vi "Field Centric Teleop Emulator.vi"(10 "Current Heading":dbl, 11 "device ID":refnum<k1>) -> (3 "Robot Velocities":T1)   [LabVIEW 2020]
uses:
  <vilib>/Analysis/NI_AALPro.lvlib
  <vilib>/Analysis/coordinate.llb/2D Cartesian Coordinate Rotation (Scalar).vi
  Drive/Implementation/Robot Velocities.ctl
panel:
  in  "Max Velocities":cluster{"vx":dbl, "vy":dbl, "w":dbl}={"vx"=10.0, "vy"=10.0, "w"=180.0}
  in  "Deadband":dbl=0.1
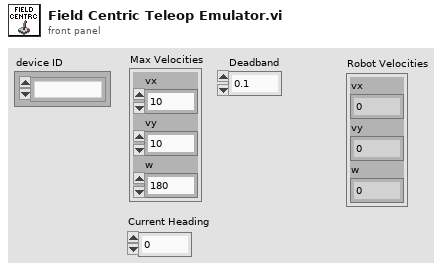
[diagram p1: front panel]
types:
  T1 = typedef "Robot Velocities.ctl" = cluster{"vx":dbl, "vy":dbl, "w":dbl}
  T2 = cluster{"X axis":i32, "Y axis":i32, "Z axis":i32, "X axis rotation":i32, "Y axis rotation":i32, "Z axis rotation":i32, "U axis":i32, "V axis":i32}
  T3 = cluster{"X axis":dbl, "Y axis":dbl, "Z axis":dbl, "X axis rotation":dbl, "Y axis rotation":dbl, "Z axis rotation":dbl, "U axis":dbl, "V axis":dbl}
  T4 = cluster{"X axis":dbl, dbl, "X axis rotation":dbl}
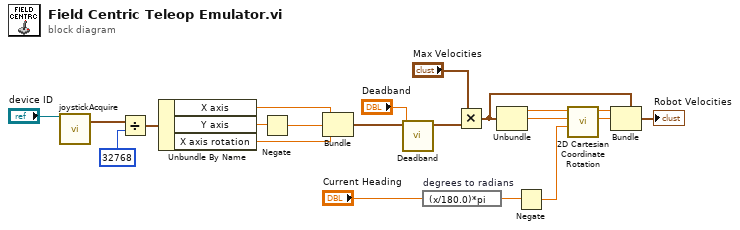
[diagram p0: block diagram]
diagram:
  n1 = call <vilib>:"joystickAcquire.vi"("device ID"="device ID") -> ("axis info"=w17:T2)  [unwired: 14 in, 4 out]
  n2 = Divide(x=w17, y=32768 ("X axis")) -> (x/y=w15:T3)
  n3 = Unbundle By Name(w15) -> ("X axis"=w13:dbl, "Y axis"=w11:dbl, "X axis rotation"=w12:dbl)
  n4 = Negate(x=w11) -> (-x=w10:dbl)
  n5 = Bundle("X axis"=w13, w10, "X axis rotation"=w12) -> (w21:T4)  [unwired: 1 in]
  n6 = call "Deadband.vi"("Deadband"="Deadband", "Robot Velocities"=w21) -> ("Adjusted Robot Velocities"=w19:T1)  [unwired: 8 in, 1 out]
  n7 = expression code="(x/180.0)*pi" "degrees to radians"("Current Heading") -> (w6:dbl)
  n8 = Multiply(x="Max Velocities", y=w19) -> (x*y=w2:T1)
  n9 = Unbundle(w2) -> ("vx"=w9:dbl, "vy"=w8:dbl)  [unwired: 1 out]
  n10 = Negate(x=w6) -> (-x=w5:dbl)
  n11 = call-poly <vilib>:"2D Cartesian Coordinate Rotation.vi"("theta"=w5, "y"=w8, "x"=w9) -> ("y out"=w3:dbl, "x out"=w4:dbl)  [unwired: 6 in, 1 out]
  n12 = Bundle(cluster=w2, "vx"=w4, "vy"=w3) -> (→"Robot Velocities":T1)  [unwired: 1 in]
